vi "Trim-Array.vi"(10 "length":i32, 11 "Array in":dbl[](array[numeric])) -> (3 "Array out":dbl[](array[numeric]))   [LabVIEW 2017]
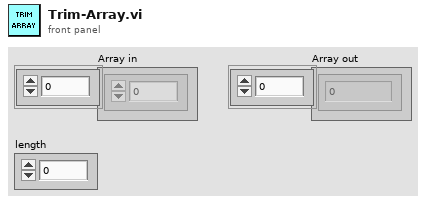
[diagram p1: front panel]
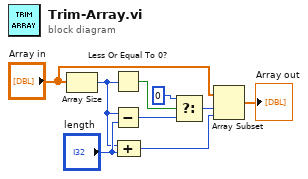
[diagram p0: block diagram]
diagram:
  n1 = Array Size(array="Array in") -> (size(s)=w6:i32)
  n2 = Less Or Equal To 0?(x=w6) -> (x <= 0?=w4:bool)
  n3 = Subtract(x=w6, y="length") -> (x-y=w8:i32)
  n4 = Compound Arithmetic op=ADD(w6, "length") -> (w3:i32)
  n5 = Select(t=0 ("length"), s=w4, f=w8) -> (s? t:f=w9:i32)
  n6 = Array Subset(array="Array in", index=w9, length=w3) -> (→"Array out":dbl[])
